vi "CloseVi (SubVI).vi"(11 "VI in":refnum<vi>) -> ()   [LabVIEW 2017]
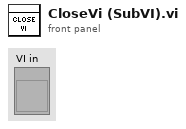
[diagram p1: front panel]
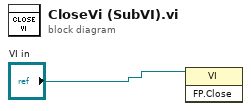
[diagram p0: block diagram]
diagram:
  n1 = invoke class="VI" method="FP.Close"(reference="VI in") -> ()  [unwired: 2 in, 3 out]
